vi "EnumToString.vi"(11 "Enum":variant) -> (3 "String":string)   [LabVIEW 2018]
uses:
  <vilib>/Utility/Data Type/NI_Data Type.lvlib
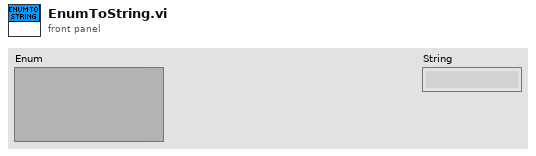
[diagram p1: front panel]
types:
  T1 = typedef "NI_Data Type.lvlib/Data Type.ctl" = enum8{"Invalid Type", "Void", "I8", "I16", "I32", "I64", "U8", "U16", "U32", "U64", "Single Float", "Double Float", "Extended Float", "Single Complex", "Double Complex", "Extended Complex", "Enum U8", "Enum U16", "Enum U32", "Enum U64", "Single Float With Unit", "Double Float With Unit", "Extended Float With Unit", "Single Complex with Unit", "Double Complex with Unit", "Extended Complex with Unit", "Boolean", "String", "Path", "Picture", "Tag", "Array", "Cluster", "Variant", "LV Variant", "Waveform", "Timestamp", "Digital Waveform", "Digital Data", "ExpressData", "Refnum", "External Data", "VI", "Poly VI", "LabVIEW Class Instance", "Fixed Point"}
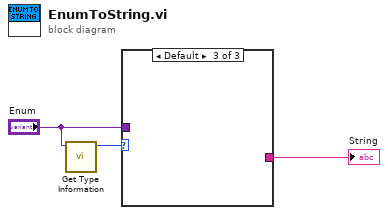
[diagram p0: block diagram]
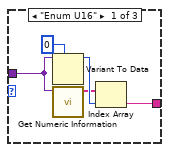
[diagram p2: hidden frame]
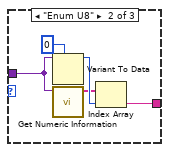
[diagram p3: hidden frame]
diagram:
  n1 = call <vilib>:"Get Type Information.vi"("Variant"="Enum") -> ("Type"=w1:T1)  [unwired: 6 in, 4 out]
  n2 = case shown="Default" w1 {
    tunnel: "Enum" -> [w6 w11 _]
    tunnel: [w4 w9 _] -> w3
    frame "Enum U16" {
      n3 = Variant To Data(type=u16 0, Variant=w6) -> (data=w8:u16)  [unwired: 1 in, 1 out]
      n4 = call <vilib>:"Get Numeric Information.vi"("Variant"=w6) -> ("Enum Names"=w7:string[])  [unwired: 7 in, 3 out]
      n5 = Index Array(array=w7, index=w8) -> (element=w4:string)
    }
    frame "Enum U8" {
      n6 = Variant To Data(type=u8 0, Variant=w11) -> (data=w13:u8)  [unwired: 1 in, 1 out]
      n7 = call <vilib>:"Get Numeric Information.vi"("Variant"=w11) -> ("Enum Names"=w12:string[])  [unwired: 7 in, 3 out]
      n8 = Index Array(array=w12, index=w13) -> (element=w9:string)
    }
    frame Default {
    }
  }
  "String" <- w3
